vi "Utility_Bool States.vi"(11 "HW_Joystick_Buttons":bool[](array[boolean])) -> (0 "Toggle On Rizing Out":bool[](array[boolean]), 1 "Falling Out":bool[](array[boolean]), 2 "Rizing Out":bool[](array[boolean]), 3 "Value Out":bool[](array[boolean]), 4 "Toggle On Falling Out":bool[](array[boolean]))   [LabVIEW 2017]
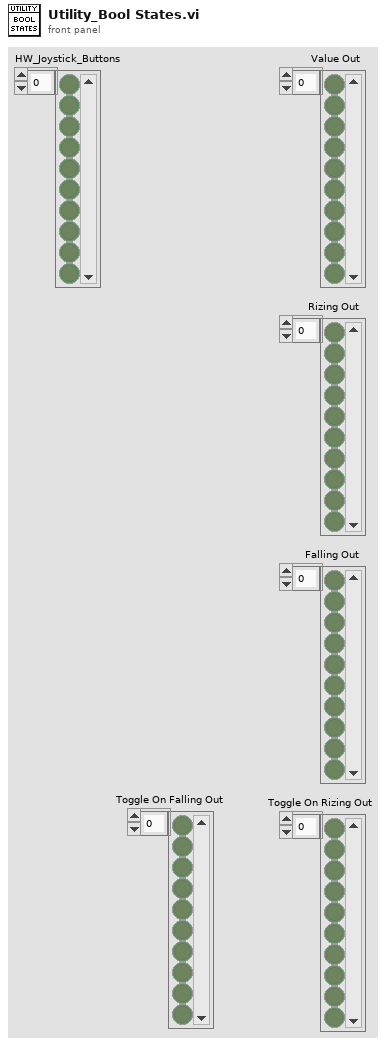
[diagram p1: front panel]
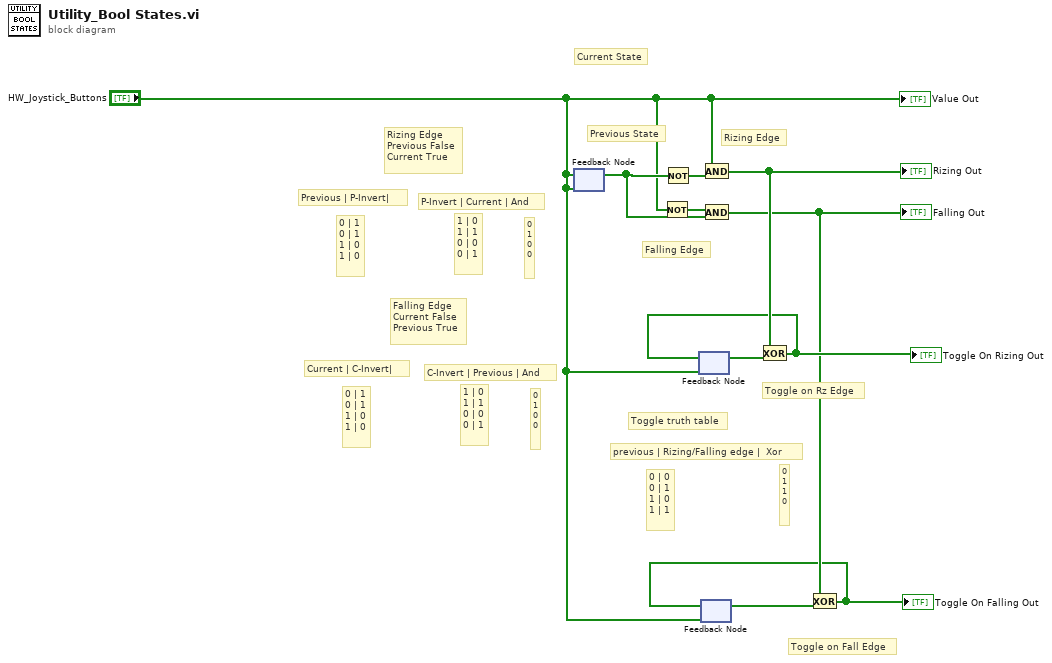
[diagram p0: block diagram]
diagram:
  # "Toggle on Fall Edge"
  # "0 | 1 \n0 | 1\n1 | 0\n1 | 0"
  # "0\n1\n0\n0"
  # "1 | 0 \n1 | 1\n0 | 0\n0 | 1"
  # "C-Invert | Previous | And"
  # "Falling Edge \nCurrent False\nPrevious True"
  # "Current | C-Invert|"
  # "0 | 1 \n0 | 1\n1 | 0\n1 | 0"
  # "0\n1\n0\n0"
  # "1 | 0 \n1 | 1\n0 | 0\n0 | 1"
  # "P-Invert | Current | And"
  # "Rizing Edge \nPrevious False\nCurrent True"
  # "Previous | P-Invert|"
  # "Toggle on Rz Edge"
  # "Toggle truth table"
  # "0\n1\n1\n0"
  # "0 | 0 \n0 | 1\n1 | 0\n1 | 1"
  # "previous | Rizing/Falling edge |  Xor"
  # "Falling Edge"
  # "Rizing Edge"
  # "Previous State"
  # "Current State"
  n1 = feedback #1("HW_Joystick_Buttons") -> (w9:bool[])
  n2 = feedback-in #1("HW_Joystick_Buttons") -> ()
  n3 = Not(x="HW_Joystick_Buttons") -> (.not. x?=w10:bool[])
  n4 = Not(x=w9) -> (.not. x?=w7:bool[])
  n5 = feedback #2("HW_Joystick_Buttons") -> (w8:bool[])
  n6 = feedback #3("HW_Joystick_Buttons") -> (w4:bool[])
  n7 = And(x="HW_Joystick_Buttons", y=w7) -> (x .and. y?=w6:bool[])
  "Rizing Out" <- w6
  n8 = And(x=w10, y=w9) -> (x .and. y?=w2:bool[])
  "Falling Out" <- w2
  n9 = Exclusive Or(1:w8, 2:w6) -> (0:w5:bool[])
  "Toggle On Rizing Out" <- w5
  n10 = feedback-in #2(w5) -> ()
  n11 = Exclusive Or(1:w4, 2:w2) -> (0:w1:bool[])
  "Toggle On Falling Out" <- w1
  n12 = feedback-in #3(w1) -> ()
  "Value Out" <- "HW_Joystick_Buttons"
